vi "PatternRecognition.vi"(7 "error in (no error)":errorcluster, 8 "MatchParameters":T1={"Number of Matches Requested"=1, "Minimum Match Score"=950.0, "Angle Ranges"=[{"Start Angle"=0.0, "End Angle"=0.0}]}, 9 "ImageIn":T3(plugin-control), 10 "TemplateFileName":string) -> (0 "error out":errorcluster, 1 "AllMatches":T2(array[cluster]) {"Bounding Box"."y" format="%.2f"; "Bounding Box"."x" format="%.2f"; "Score" format="%.2f"; "Scale" format="%.2f"; "Angle" format="%.2f"; "Position"."y" format="%.2f"; "Position"."x" format="%.2f"}, 2 "Position":cluster{"x":sgl, "y":sgl}, 3 "ImageFoundPattern":T3(plugin-control), 4 "Number of Matches":i32)   [LabVIEW 2021]
uses:
  <vilib>/vision/NI_Vision_Development_Module.lvlib
panel:
  out "Template":T3(plugin-control)
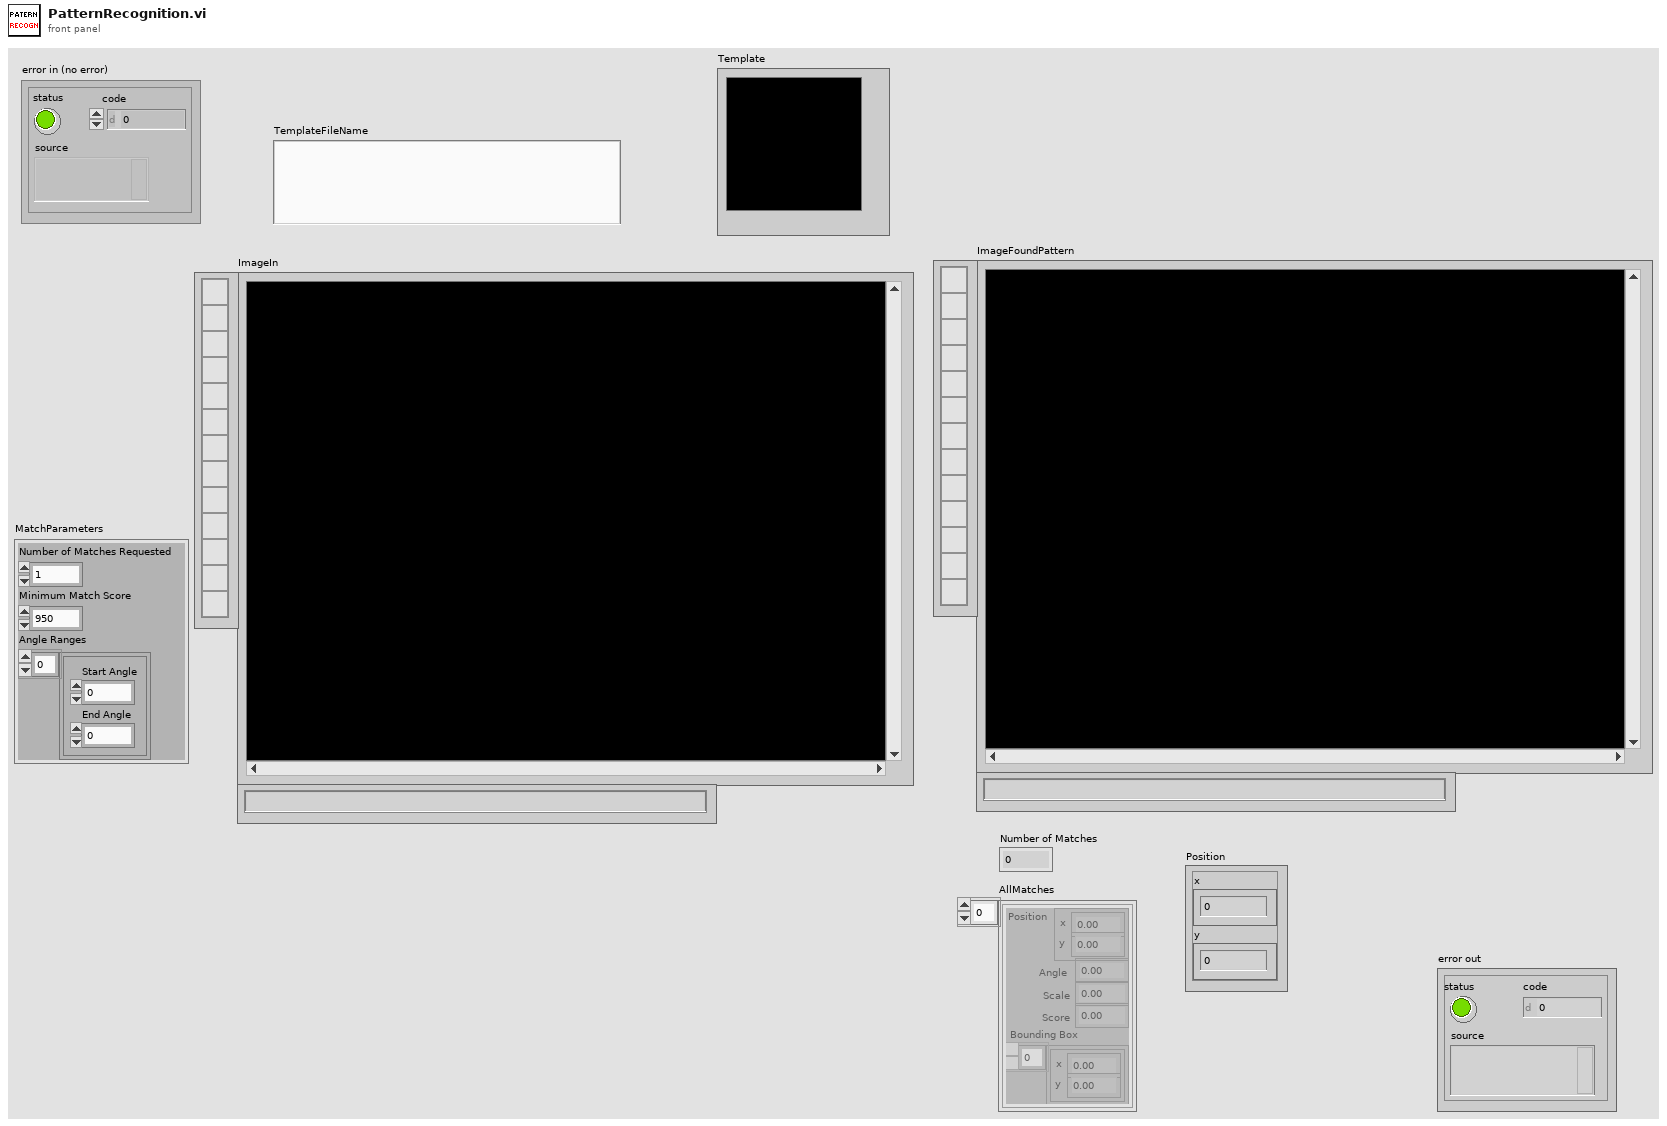
[diagram p1: front panel]
types:
  T1 = cluster{"Number of Matches Requested":i32, "Minimum Match Score":sgl, "Angle Ranges":cluster{"Start Angle":sgl, "End Angle":sgl}[]}
  T2 = cluster{"Position":cluster{"x":sgl, "y":sgl}, "Angle":sgl, "Scale":sgl, "Score":sgl, "Bounding Box":cluster{"x":sgl, "y":sgl}[]}[]
  T3 = typedef "IMAQ Image.ctl" = refnum<image>
  T4 = typedef "Image Type" = u32
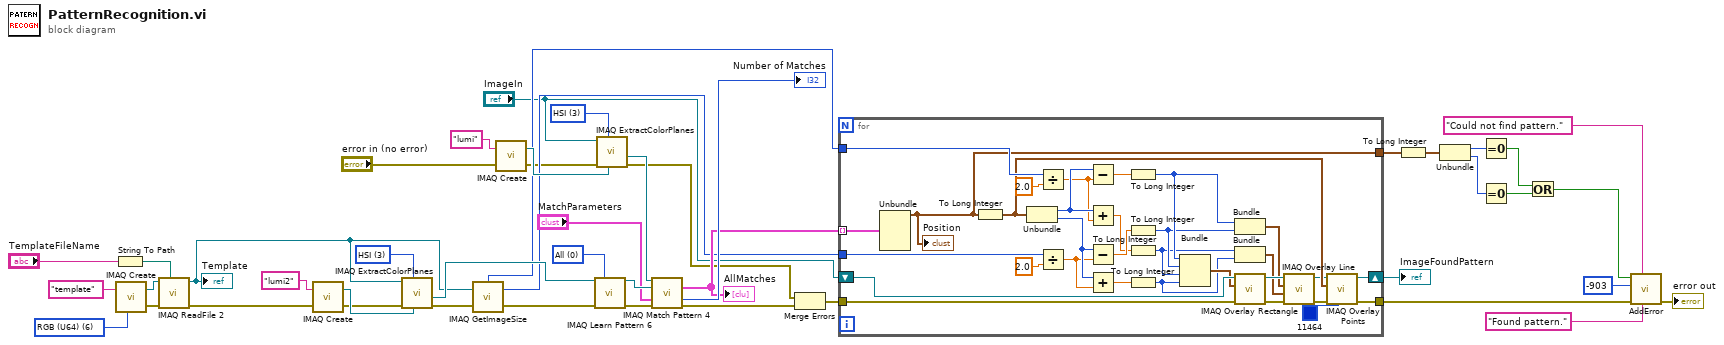
[diagram p0: block diagram]
diagram:
  w34 = u16 3 items=["RGB", "HSL", "HSV", "HSI"] ("Color Mode")
  w40 = u16 3 items=["RGB", "HSL", "HSV", "HSI"] ("Color Mode")
  w42 = 0 items=["All", "Low Discrepancy Sampling", "Grayscale Value Pyramid", "Gradients Pyramid"] ("Algorithm")
  w44 = T4 6 items=["Grayscale (U8)", "Grayscale (I16)", "Grayscale (SGL)", "Complex (CSG)", "RGB (U32)", "HSL (U32)", "RGB (U64)", "Grayscale (U16)"] ("Image Type")
  n1 = String To Path(string="TemplateFileName") -> (path=w14:path)
  n2 = call "IMAQ Create"("Image Name"="template", "Image Type"=w44) -> ("New Image"=w46:T3, "error out"=w43:errorcluster)  [unwired: 3 in]
  n3 = call "IMAQ ReadFile 2"("File Path"=w14, "error in (no error)"=w43, "Image"=w46) -> ("error out"=w24:errorcluster, "Image Out"=w28:T3)  [unwired: 4 in, 3 out]
  "Template" <- w28
  n4 = call "IMAQ Create"("Image Name"="lumi2", "error in (no error)"=w24) -> ("New Image"=w32:T3, "error out"=w23:errorcluster)  [unwired: 2 in, 1 out]
  n5 = call "IMAQ ExtractColorPlanes"("Blue or Luma or Val or Inten Plane"=w32, "Color Mode"=w34, "error in (no error)"=w23, "Image Src"=w28) -> ("error out"=w22:errorcluster, "Blue or Luma or Val or Inten Plane out"=w33:T3)  [unwired: 4 in, 2 out]
  n6 = call "IMAQ GetImageSize"("Image"=w28, "error in (no error)"=w22) -> ("Y Resolution"=w26:i32, "X Resolution"=w27:i32, "error out"=w21:errorcluster)  [unwired: 2 in]
  n7 = call "IMAQ Create"("Image Name"="lumi", "error in (no error)"="error in (no error)") -> ("New Image"=w38:T3, "error out"=w25:errorcluster)  [unwired: 2 in, 1 out]
  n8 = call "IMAQ Learn Pattern 6"("Image"=w33, "Algorithm"=w42, "error in (no error)"=w21) -> ("Template Image Out"=w37:T3, "error out"=w36:errorcluster)  [unwired: 10 in, 1 out]
  n9 = call "IMAQ ExtractColorPlanes"("Blue or Luma or Val or Inten Plane"=w38, "Color Mode"=w40, "error in (no error)"=w25, "Image Src"="ImageIn") -> ("error out"=w20:errorcluster, "Blue or Luma or Val or Inten Plane out"=w31:T3)  [unwired: 4 in, 2 out]
  n10 = call "IMAQ Match Pattern 4"("Image"=w31, "Template Image"=w37, "Parameters"="MatchParameters", "error in (no error)"=w36) -> ("Matches (pixel)"=w29:T2, "Number of Matches"=→"Number of Matches":i32, "error out"=w19:errorcluster)  [unwired: 7 in, 2 out]
  "AllMatches" <- w29
  n11 = Merge Errors(w20, w19) -> (w15:errorcluster)
  n12 = for {
    shift-right: [w62] -> w30
    shift-left: "ImageIn" -> [w77]
    tunnel: w29 -> [w76] mode=indexing
    tunnel: w27 -> [w74]
    tunnel: w26 -> [w72]
    tunnel: w15 -> [w60]
    tunnel: [w59] -> w4
    tunnel: [w58] -> w12
    n13 = Unbundle(w76) -> ("Position"=w58:cluster{"x":sgl, "y":sgl})  [unwired: 4 out]
    "Position" <- w58
    n14 = To Long Integer(number=w58) -> (32bit integer=w61:cluster{"x":i32, "y":i32})
    n15 = Unbundle(w61) -> ("x"=w68:i32, "y"=w66:i32)
    n16 = Divide(x=w74, y=2.0) -> (x/y=w67:dbl)
    n17 = Divide(x=w72, y=2.0) -> (x/y=w65:dbl)
    n18 = Subtract(x=w68, y=w67) -> (x-y=w71:dbl)
    n19 = Add(x=w68, y=w67) -> (x+y=w64:dbl)
    n20 = Subtract(x=w66, y=w65) -> (x-y=w70:dbl)
    n21 = Add(x=w66, y=w65) -> (x+y=w69:dbl)
    n22 = To Long Integer(number=w71) -> (32bit integer=w56:i32)
    n23 = To Long Integer(number=w70) -> (32bit integer=w55:i32)
    n24 = To Long Integer(number=w64) -> (32bit integer=w53:i32)
    n25 = To Long Integer(number=w69) -> (32bit integer=w52:i32)
    n26 = Bundle(w56, w55, w53, w52) -> (w63:cluster{i32, i32, i32, i32})  [unwired: 1 in]
    n27 = Bundle(w56, w55) -> (w54:cluster{i32, i32})  [unwired: 1 in]
    n28 = Bundle(w53, w52) -> (w51:cluster{i32, i32})  [unwired: 1 in]
    n29 = call "IMAQ Overlay Rectangle"("error in (no error)"=w60, "Rectangle"=w63, "Image"=w77) -> ("error out"=w50:errorcluster, "Image Out"=w57:T3)  [unwired: 7 in]
    n30 = call "IMAQ Overlay Line"("error in (no error)"=w50, "End Point"=w51, "Start Point"=w54, "Image"=w57) -> ("error out"=w49:errorcluster, "Image Out"=w48:T3)  [unwired: 6 in]
    n31 = call "IMAQ Overlay Points"("Color"=u32 11464, "error in (no error)"=w49, "Point"=w61, "Image"=w48) -> ("error out"=w59:errorcluster, "Image Out"=w62:T3)  [unwired: 6 in]
  }
  "ImageFoundPattern" <- w30
  n32 = To Long Integer(number=w12) -> (32bit integer=w11:cluster{"x":i32, "y":i32})
  n33 = Unbundle(w11) -> ("x"=w10:i32, "y"=w9:i32)
  n34 = Equal To 0?(x=w10) -> (x = 0?=w8:bool)
  n35 = Equal To 0?(x=w9) -> (x = 0?=w7:bool)
  n36 = Or(x=w8, y=w7) -> (x .or. y?=w6:bool)
  n37 = call "AddError.vi"("NoErrorMessage"="Found pattern.", "ErrorMessage"="Could not find pattern.", "error in"=w4, "code"=-903, "Error?"=w6) -> ("Error out"=→"error out":errorcluster)  [unwired: 6 in]
